vi "Plot Helper (Vector).vi"(8 "error in (no error)":errorcluster, 9 "offset vector":sgl[](array[numeric]), 10 "x vector":sgl[](array[numeric])) -> (0 "error out":errorcluster, 3 "3D Plot lvclass Array out":refnum<class "3D Plot Datatype.lvclass">[](array[class]))   [LabVIEW 2020, in "3D Pie Datatype.lvclass"]
doc: "Generates a pie chart."
uses:
  <vilib>/Math Plots/3D Math Plots/3D Pie/3D Pie Datatype/3D Pie Datatype.lvclass
  <vilib>/Math Plots/3D Math Plots/3D Plot/3D Plot Datatype/3D Plot Datatype.lvclass
  e:/builds/penguin/labview/branches/2020/dev/dist/vi.lib/Math Plots/3D Math Plots/3D Plot/3D Plot Datatype/3D Plot Datatype.lvclass
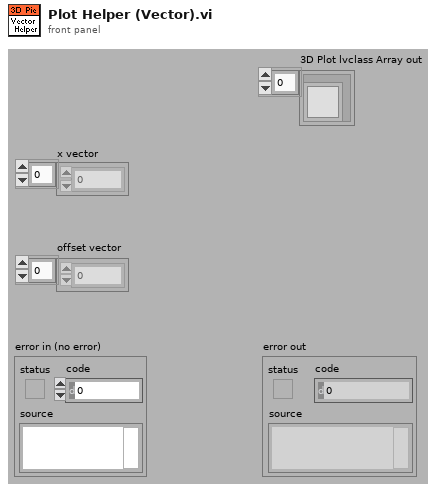
[diagram p1: front panel]
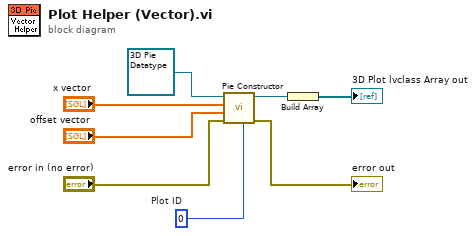
[diagram p0: block diagram]
diagram:
  w5 = 0  # Plot ID
  n1 = call <vilib>:"Pie Constructor.vi"("Plot ID"=w5, "error in (no error)"="error in (no error)", "offset vector"="offset vector", "x vector"="x vector", "3D Quiver Datatype.lvclass in"=refnum<class "3D Pie Datatype.lvclass"> refnum) -> ("error out"=→"error out":errorcluster, "3D Quiver Datatype.lvclass out"=w4:refnum<class "3D Pie Datatype.lvclass">)  [unwired: 5 out]
  n2 = Build Array(w4) -> (→"3D Plot lvclass Array out":refnum<class "3D Pie Datatype.lvclass">[])
